vi "Drive Controller.vi"(8 "error in":errorcluster) -> ()   [LabVIEW 2019]
doc: "This VI executes continuously carrying out the current operation and responding to updates or new operation requests. It will often contain the timing or control code that is difficult to place directly in TeleOp. This VI generally opens all sensors and motors and isolates the rest of the robot code from knowing implementation details of how the operations are carried out."
uses:
  <vilib>/Rock Robotics/WPI/Framework/Completion Status.ctl
  Drive Setpoints.ctl
  Drive Operations.ctl
  <vilib>/Rock Robotics/WPI/ThirdParty/Phoenix-LabVIEW/Motor Controller/Controls/CTRE_Phoenix_MotorControl_ControlMode.ctl
  <vilib>/Rock Robotics/WPI/ThirdParty/Phoenix-LabVIEW/Motor Controller/Get/CTRE_Phoenix_MotorController_GetSelectedSensorData.vi
  <vilib>/Rock Robotics/WPI/SafetyOutput/WPI_SafetyOutputConfigMenu.ctl
  <vilib>/Rock Robotics/WPI/RobotDrive/WPI_RobotDriveOpen2MotorWithExistingMotors.vi
panel:
  in  "Interactive Values":T1
  in  "Buttons":cluster{"Execute Cmd":bool, "Abort Cmd":bool}
  out "Command Timing":cluster{"Start Time (ms)":u32, "Iterations":i32}
  out "Status":T3
  out "Current\nCmd":string
  # "Tip: The graph shows the motor setpoints. It may also be helpful to observe inputs and sensor values.\nYou may also want to display tuning or debugging controls."
  # "Interactive Command: You may fill in the settings for a command\nand schedule it with the Execute button. You can observe and abort\nany command while fine tuning the code for the controller."
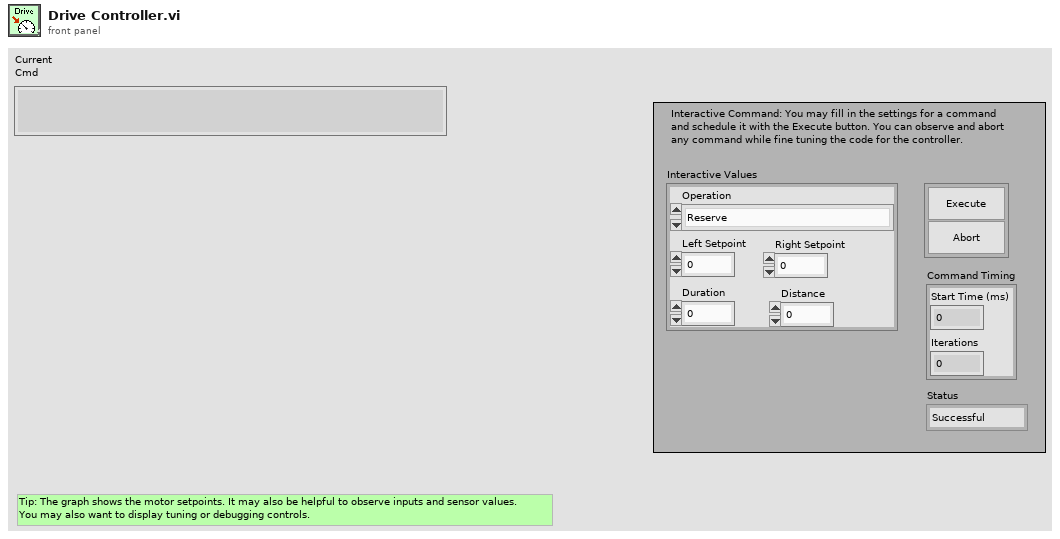
[diagram p1: front panel]
types:
  T1 = typedef "Drive Setpoints.ctl" = cluster{"Operation":T2, "Left Setpoint":dbl, "Right Setpoint":dbl, "Duration":dbl, "Distance":dbl}
  T2 = typedef "Drive Operations.ctl" = enum16{"Reserve", "Read Current", "Immediate", "Drive for Time", "Drive for Distance", "Turn angle"}
  T3 = typedef "Completion Status.ctl" = enum16{"Successful", "Aborted", "Incomplete"}
  T4 = typedef "WPI_SafetyOutputConfigMenu.ctl" = enum16{"Enable", "Disable"}
  T5 = typedef "WPI_MotorControlDeviceRef.ctl" = cluster{"DeviceStatus":errorcluster, "Type":T6, "PWM":cluster{"PWM Channel":T7, "DeadBand":T8}, "CAN":cluster{"Device Number":u8, "SetOutput VI Ref":variant, "GetOutput VI Ref":variant, "Enable VI Ref":variant, "Disable VI Ref":variant, "Data":variant}, "Invert":bool, "DIO PWM":cluster{"PWM \"Enable\" Channel":T7, "DIOChannel":T9, "PWM Rate":dbl}}
  T6 = typedef "WPI_MotorControlType.ctl" = enum16{"PWM", "CAN", "DIO PWM"}
  T7 = typedef "FPGA_DIOPWMChannel.ctl" = enum8{"PWM 0", "PWM 1", "PWM 2", "PWM 3", "PWM 4", "PWM 5", "PWM 6", "PWM 7", "PWM 8", "PWM 9", "PWM MXP 0", "PWM MXP 1", "PWM MXP 2", "PWM MXP 3", "PWM MXP 4", "PWM MXP 5", "PWM MXP 6", "PWM MXP 7", "PWM MXP 8", "PWM MXP 9", "Invalid"}
  T8 = typedef "WPI_PWMDeadband.ctl" = cluster{"Name":string, "maxPositivePwm":i32, "minPositivePwm":i32, "centerPwm":i32, "maxNegativePwm":i32, "minNegativePwm":i32, "angularRange":u16}
  T9 = typedef "FPGA_DIOChannel.ctl" = enum8{"DIO 0", "DIO 1", "DIO 2", "DIO 3", "DIO 4", "DIO 5", "DIO 6", "DIO 7", "DIO 8", "DIO 9", "DIO MXP 0", "DIO MXP 1", "DIO MXP 2", "DIO MXP 3", "DIO MXP 4", "DIO MXP 5", "DIO MXP 6", "DIO MXP 7", "DIO MXP 8", "DIO MXP 9", "DIO MXP 10", "DIO MXP 11", "DIO MXP 12", "DIO MXP 13", "DIO MXP 14", "DIO MXP 15", "SPI Port CS1", "SPI Port CS2", "SPI Port CS3", "SPI Port MISO", "SPI Port MOSI", "Invalid"}
  T10 = typedef "WPI_RobotDriveDevRef.ctl" = cluster{"DevStatus":errorcluster, "Motors[]":T5[], "Square Inputs":bool, "Max Output":dbl}
  T11 = enum16{"FollowerType_PercentOutput", "FollowerType_AuxOutput1"}
  T12 = typedef "Command Status Info.ctl" = cluster{"Name":string, "Status":T3, "notifier out":T13}
  T13 = typedef "Completion Notifier.ctl" = refnum<notifier>
  T14 = cluster{"SubSystem Data":T1, cluster{"Start Time (ms)":u32, "Iterations":i32}, cluster{"Command Info":T12, "Description":string, "Default Command":T1, "queue out":refnum<queue>, "Subsystem Name":string}}
  T15 = typedef "CTRE_Phoenix_MotorControl_ControlMode.ctl" = u16
  T16 = cluster{"SubSystem Data":T1, cluster{"Start Time (ms)":u32, "Iterations":i32}, "Default Command Arguments":cluster{"Command Info":T12, "Description":string, "Default Command":T1, "queue out":refnum<queue>, "Subsystem Name":string}}
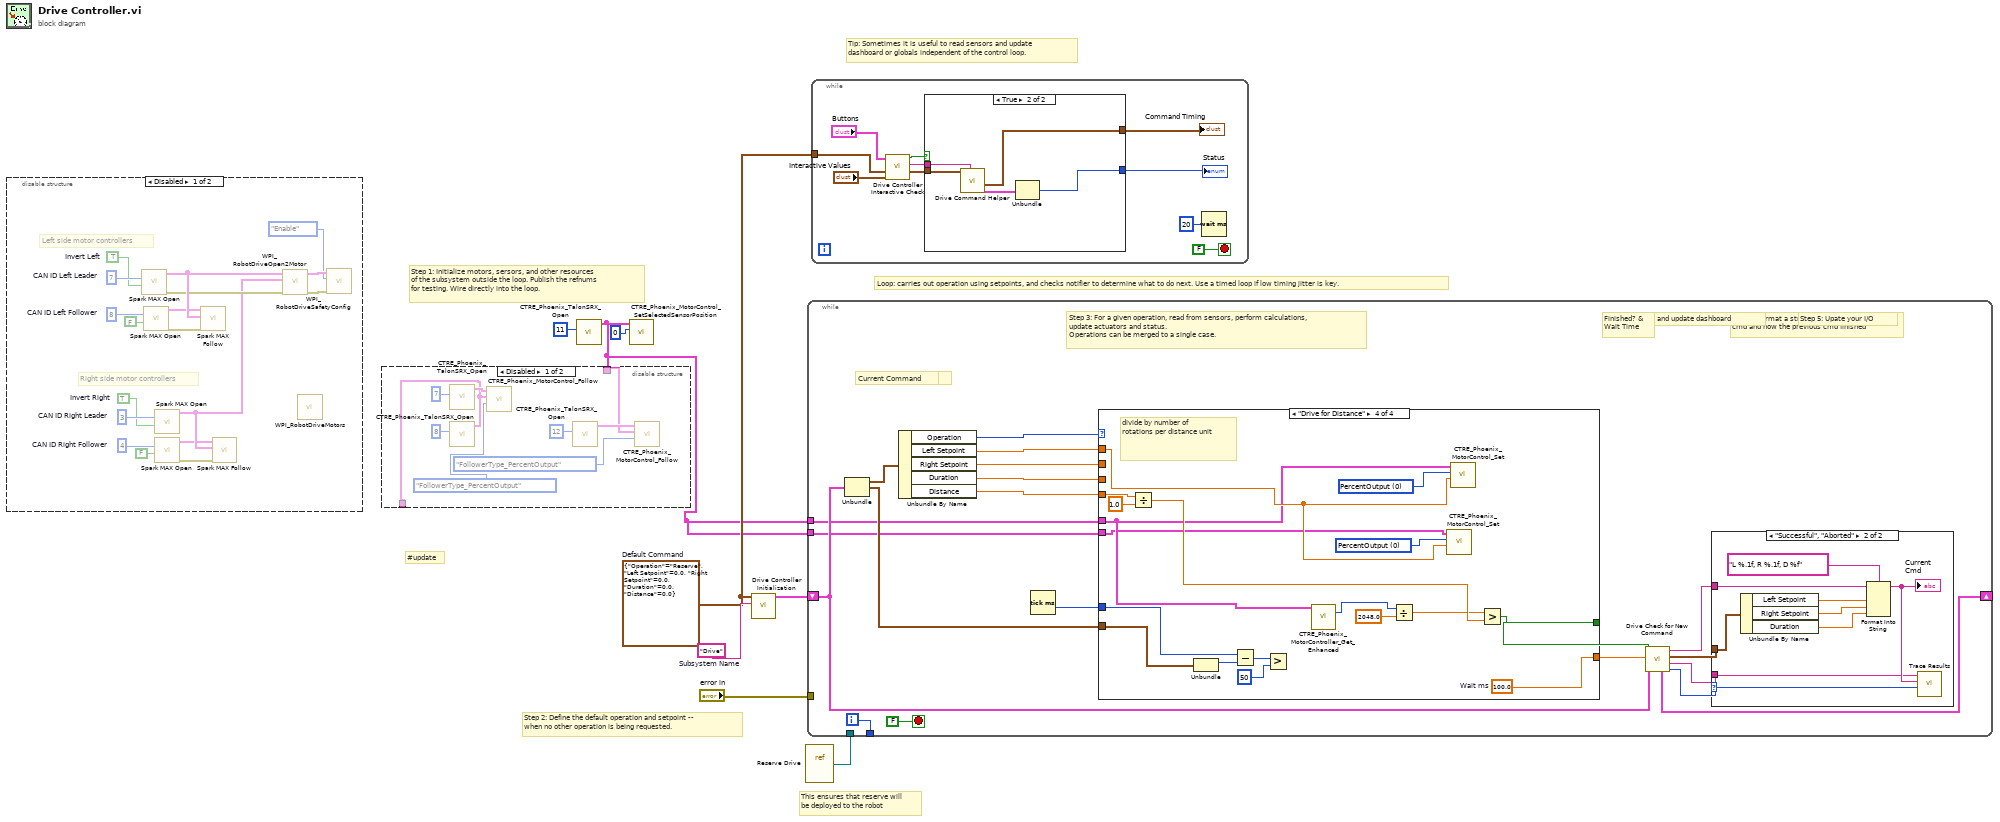
[diagram p0: block diagram]
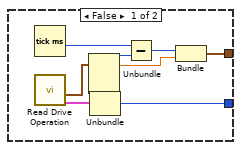
[diagram p4: hidden frame]
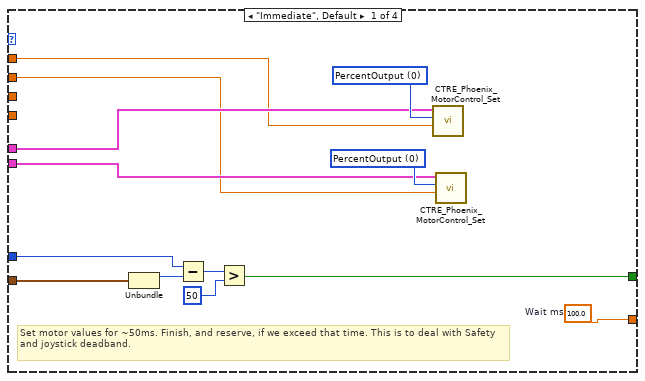
[diagram p6: hidden frame]
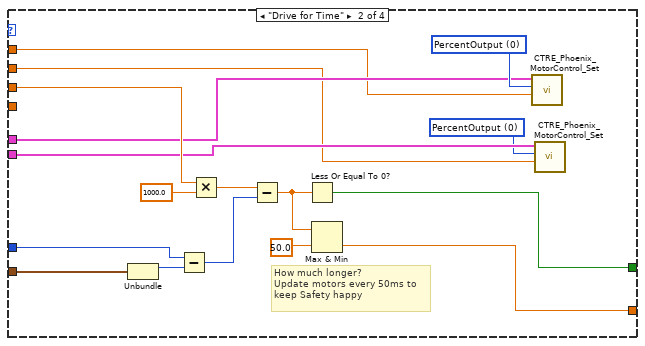
[diagram p7: hidden frame]
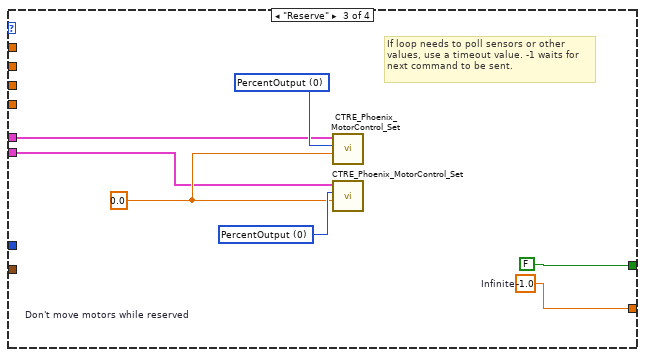
[diagram p8: hidden frame]
diagram:
  w4 = T1 {"Operation"=enum."Reserve", "Left Setpoint"=0.0, "Right Setpoint"=0.0, "Duration"=0.0, "Distance"=0.0}  # Default Command
  w8 = "Drive"  # Subsystem Name
  # "#update"
  # "This ensures that reserve will\nbe deployed to the robot"
  # "Tip: Sometimes it is useful to read sensors and update\ndashboard or globals independent of the control loop."
  # "Step 2: Define the default operation and setpoint --\nwhen no other operation is being requested."
  # "Step 1: Initialize motors, sersors, and other resources\nof the subsystem outside the loop. Publish the refnums\nfor testing. Wire directly into the loop."
  # "Loop: carries out operation using setpoints, and checks notifier to determine what to do next. Use a timed loop if low timing jitter is key."
  n1 = disable-structure shown="Disabled" {
    frame Disabled {
      w15 = TRUE  # Invert Left
      w14 = TRUE  # Invert Right
      w20 = u8 3  # CAN ID Right Leader
      w19 = u8 4  # CAN ID Right Follower
      w26 = u8 7  # CAN ID Left Leader
      w27 = u8 8  # CAN ID Left Follower
      # "Right side motor controllers"
      # "Left side motor controllers"
      n2 = call <vilib>:"Spark MAX Open.vi"("Invert"=w15, "Device Number"=w26) -> ("error out"=w24:errorcluster, "MotorControlDeviceRef"=w25:T5)  [unwired: 8 in]
      n3 = call <vilib>:"Spark MAX Open.vi"("Invert"=FALSE, "Device Number"=w27) -> ("error out"=w22:errorcluster, "MotorControlDeviceRef"=w23:T5)  [unwired: 8 in]
      n4 = call <vilib>:"Spark MAX Open.vi"("Invert"=w14, "Device Number"=w20) -> ("MotorControlDeviceRef"=w11:T5)  [unwired: 8 in, 1 out]
      n5 = call <vilib>:"Spark MAX Open.vi"("Invert"=FALSE, "Device Number"=w19) -> ("error out"=w21:errorcluster, "MotorControlDeviceRef"=w9:T5)  [unwired: 8 in]
      n6 = call <vilib>:"Spark MAX Follow.vi"("error in (no error)"=w22, "Master Controller"=w25, "MotorControlDeviceRef"=w23) -> ()  [unwired: 7 in, 2 out]
      n7 = call <vilib>:"Spark MAX Follow.vi"("error in (no error)"=w21, "Master Controller"=w11, "MotorControlDeviceRef"=w9) -> ()  [unwired: 7 in, 2 out]
      n8 = call-poly <vilib>:"WPI_RobotDriveOpen2Motor.vi"("error in (no error)"=w24, "Right Motor Dev Ref"=w11, "Left Motor Dev Ref"=w25) -> ("error out"=w17:errorcluster, "RobotDriveDevRef"=w18:T10)  [unwired: 7 in]
      n9 = call <vilib>:"WPI_RobotDriveMotors.vi"() -> ()  [unwired: 4 in, 8 out]
      n10 = call <vilib>:"WPI_RobotDriveSafetyConfig.vi"("error in (no error)"=w17, "mode"=WPI_SafetyOutputConfigMenu."Enable", "RobotDriveDevRef"=w18) -> ("RobotDriveDevRef"=w10:T10)  [unwired: 7 in, 1 out]
    }
    frame Enabled {
    }
  }
  n11 = call <vilib>:"CTRE_Phoenix_TalonSRX_Open.vi"("Device Number"=u8 11) -> ("CAN Talon SRX Ref"=w1:T5)  [unwired: 9 in, 1 out]
  n12 = disable-structure shown="Disabled" {
    disable-tunnel: [w30 _] -> _
    disable-tunnel: w1 -> [w29 _]
    frame Disabled {
      n13 = call <vilib>:"CTRE_Phoenix_TalonSRX_Open.vi"("Device Number"=u8 7) -> ("CAN Talon SRX Ref"=w31:T5)  [unwired: 9 in, 1 out]
      n14 = call <vilib>:"CTRE_Phoenix_TalonSRX_Open.vi"("Device Number"=u8 8) -> ("CAN Talon SRX Ref"=w30:T5)  [unwired: 9 in, 1 out]
      n15 = call <vilib>:"CTRE_Phoenix_MotorControl_Follow.vi"("FollowerType"=T11."FollowerType_PercentOutput", "Master Controller to Follow"=w30, "PhoenixMotorControlDevRef"=w31) -> ()  [unwired: 7 in, 2 out]
      n16 = call <vilib>:"CTRE_Phoenix_TalonSRX_Open.vi"("Device Number"=u8 12) -> ("CAN Talon SRX Ref"=w36:T5)  [unwired: 9 in, 1 out]
      n17 = call <vilib>:"CTRE_Phoenix_MotorControl_Follow.vi"("FollowerType"=T11."FollowerType_PercentOutput", "Master Controller to Follow"=w29, "PhoenixMotorControlDevRef"=w36) -> ()  [unwired: 7 in, 2 out]
    }
    frame Enabled {
    }
  }
  n18 = call <vilib>:"CTRE_Phoenix_MotorControl_SetSelectedSensorPosition.vi"("New Sensor Position"=0, "PhoenixMotorControlDevRef"=w1) -> ()  [unwired: 8 in, 2 out]
  n19 = call "Drive Controller Initialization.vi"("Subsystem Name"=w8, "Default Command"=w4) -> ("Current Command"=w6:T14)  [unwired: 9 in]
  n20 = vi-ref "Reserve Drive.vi"() -> (w5:refnum<vi>)
  n21 = while {
    shift-right: [w47] -> _
    shift-left: w6 -> [w40]
    tunnel: [w55] -> _
    tunnel: "error in" -> [_]
    tunnel: w5 -> [_]
    tunnel: w1 -> [w38]
    tunnel: w1 -> [w37]
    i -> [w55]
    stop <- FALSE stop-if-true
    # "Step 5: Upate your I/O"
    # "Step 4: Format a string to describe this\ncmd and how the previous cmd finished"
    # "Current Command"
    # "Update motors and update dashboard"
    # "Access Cmd setpoints"
    # "Finished? &\nWait Time"
    # "Step 3: For a given operation, read from sensors, perform calculations,\nupdate actuators and status.\nOperations can be merged to a single case."
    n22 = Unbundle(w40) -> ("SubSystem Data"=w54:T1, w41:cluster{"Start Time (ms)":u32, "Iterations":i32})  [unwired: 1 out]
    n23 = Unbundle By Name(w54) -> ("Operation"=w53:T2, "Left Setpoint"=w52:dbl, "Right Setpoint"=w51:dbl, "Duration"=w50:dbl, "Distance"=w39:dbl)
    n24 = Tick Count (ms)() -> (millisecond timer value=w49:u32)
    n25 = case shown="\"Drive for Distance\"" w53 {
      tunnel: [w78 w85 w102 w115] -> w46
      tunnel: [w73 w90 FALSE ("ignore previous (F)") w105] -> w45
      tunnel: w41 -> [w72 w92 _ w114]
      tunnel: w52 -> [w67 w81 _ w111]
      tunnel: w51 -> [w66 w80 _ _]
      tunnel: w50 -> [_ w89 _ _]
      tunnel: w49 -> [w74 w88 _ w112]
      tunnel: w39 -> [_ _ _ w120]
      tunnel: w38 -> [w68 w82 w96 w103]
      tunnel: w37 -> [w69 w83 w97 w104]
      frame "Immediate", Default {
        w70 = T15 0 items=["PercentOutput"=0, "Position"=1, "Velocity"=2, "Current"=3, "Follower"=5, "MotionProfile"=6, "MotionMagic"=7, "MotionProfileArc"=10, "Disabled"=15] ("Control Mode")
        w71 = T15 0 items=["PercentOutput"=0, "Position"=1, "Velocity"=2, "Current"=3, "Follower"=5, "MotionProfile"=6, "MotionMagic"=7, "MotionProfileArc"=10, "Disabled"=15] ("Control Mode")
        w78 = 100.0  # Wait ms
        # "Set motor values for ~50ms. Finish, and reserve, if we exceed that time. This is to deal with Safety and joystick deadband."
        n26 = Unbundle(w72) -> ("Start Time (ms)"=w75:u32)  [unwired: 1 out]
        n27 = Subtract(x=w74, y=w75) -> (x-y=w76:u32)
        n28 = Greater?(x=w76, y=u8 50 ("Left Motor")) -> (0:w73:bool)
        n29 = call <vilib>:"CTRE_Phoenix_MotorControl_Set.vi"("Output"=w67, "Control Mode"=w71, "PhoenixMotorControlDevRef"=w69) -> ()  [unwired: 7 in, 2 out]
        n30 = call <vilib>:"CTRE_Phoenix_MotorControl_Set.vi"("Output"=w66, "Control Mode"=w70, "PhoenixMotorControlDevRef"=w68) -> ()  [unwired: 7 in, 2 out]
      }
      frame "Drive for Time" {
        w79 = T15 0 items=["PercentOutput"=0, "Position"=1, "Velocity"=2, "Current"=3, "Follower"=5, "MotionProfile"=6, "MotionMagic"=7, "MotionProfileArc"=10, "Disabled"=15] ("Control Mode")
        w84 = T15 0 items=["PercentOutput"=0, "Position"=1, "Velocity"=2, "Current"=3, "Follower"=5, "MotionProfile"=6, "MotionMagic"=7, "MotionProfileArc"=10, "Disabled"=15] ("Control Mode")
        # "How much longer?\nUpdate motors every 50ms to\nkeep Safety happy"
        n31 = Unbundle(w92) -> ("Start Time (ms)"=w91:u32)  [unwired: 1 out]
        n32 = Subtract(x=w88, y=w91) -> (x-y=w95:u32)
        n33 = Multiply(x=w89, y=1000.0) -> (x*y=w94:dbl)
        n34 = Subtract(x=w94, y=w95) -> (x-y=w87:dbl)
        n35 = Less Or Equal To 0?(x=w87) -> (x <= 0?=w90:bool)
        n36 = Max & Min(x=w87, y=50.0) -> (min(x,y)=w85:dbl)  [unwired: 1 out]
        n37 = call <vilib>:"CTRE_Phoenix_MotorControl_Set.vi"("Output"=w81, "Control Mode"=w84, "PhoenixMotorControlDevRef"=w83) -> ()  [unwired: 7 in, 2 out]
        n38 = call <vilib>:"CTRE_Phoenix_MotorControl_Set.vi"("Output"=w80, "Control Mode"=w79, "PhoenixMotorControlDevRef"=w82) -> ()  [unwired: 7 in, 2 out]
      }
      frame "Reserve" {
        w99 = T15 0 items=["PercentOutput"=0, "Position"=1, "Velocity"=2, "Current"=3, "Follower"=5, "MotionProfile"=6, "MotionMagic"=7, "MotionProfileArc"=10, "Disabled"=15] ("Control Mode")
        w100 = T15 0 items=["PercentOutput"=0, "Position"=1, "Velocity"=2, "Current"=3, "Follower"=5, "MotionProfile"=6, "MotionMagic"=7, "MotionProfileArc"=10, "Disabled"=15] ("Control Mode")
        w98 = 0.0  # Don't move motors while reserved
        w102 = -1.0  # Infinite
        # "If loop needs to poll sensors or other\nvalues, use a timeout value. -1 waits for\nnext command to be sent."
        n39 = call <vilib>:"CTRE_Phoenix_MotorControl_Set.vi"("Output"=w98, "Control Mode"=w100, "PhoenixMotorControlDevRef"=w97) -> ()  [unwired: 7 in, 2 out]
        n40 = call <vilib>:"CTRE_Phoenix_MotorControl_Set.vi"("Output"=w98, "Control Mode"=w99, "PhoenixMotorControlDevRef"=w96) -> ()  [unwired: 7 in, 2 out]
      }
      frame "Drive for Distance" {
        w107 = T15 0 items=["PercentOutput"=0, "Position"=1, "Velocity"=2, "Current"=3, "Follower"=5, "MotionProfile"=6, "MotionMagic"=7, "MotionProfileArc"=10, "Disabled"=15] ("Control Mode")
        w110 = T15 0 items=["PercentOutput"=0, "Position"=1, "Velocity"=2, "Current"=3, "Follower"=5, "MotionProfile"=6, "MotionMagic"=7, "MotionProfileArc"=10, "Disabled"=15] ("Control Mode")
        w115 = 100.0  # Wait ms
        # "divide by number of rotations per distance unit"
        n41 = Divide(x=w120, y=1.0) -> (x/y=w119:dbl)
        n42 = Unbundle(w114) -> ("Start Time (ms)"=w113:u32)  [unwired: 1 out]
        n43 = Subtract(x=w112, y=w113) -> (x-y=w116:u32)
        n44 = Greater?(x=w116, y=u8 50 ("Left Motor")) -> ()  [unwired: 1 out]
        n45 = call-poly <vilib>:"CTRE_Phoenix_MotorController_Get_Enhanced.vi"("PhoenixMotorControlDevRef"=w104) -> ("Position (Raw Sensor Units)"=w106:i32)  [unwired: 11 in, 3 out]
        n46 = Divide(x=w106, y=2048.0) -> (x/y=w109:dbl)
        n47 = call <vilib>:"CTRE_Phoenix_MotorControl_Set.vi"("Output"=w111, "Control Mode"=w110, "PhoenixMotorControlDevRef"=w103) -> ()  [unwired: 7 in, 2 out]
        n48 = call <vilib>:"CTRE_Phoenix_MotorControl_Set.vi"("Output"=w111, "Control Mode"=w107, "PhoenixMotorControlDevRef"=w104) -> ()  [unwired: 7 in, 2 out]
        n49 = Greater?(x=w109, y=w119) -> (0:w105:bool)
      }
    }
    n50 = call "Drive Check for New Command.vi"("input cluster"=w40, "Wait time (ms)"=w46, "Finished?"=w45) -> ("Completion"=w48:T3, "Subsystem Name"=w42:string, "Current Command"=w43:T1, "Initial Trace String"=w44:string, "Next Command"=w47:T16)  [unwired: 4 in]
    n51 = case shown="\"Successful\", \"Aborted\"" w48 {
      selector: w48 -> [_ w65]
      tunnel: w44 -> [_ w60]
      tunnel: w43 -> [_ w61]
      tunnel: w42 -> [_ w57]
      frame "Incomplete", Default {
        # "Continuing current command"
      }
      frame "Successful", "Aborted" {
        # "Report and setup for next command"
        n52 = Unbundle By Name(w61) -> ("Left Setpoint"=w63:dbl, "Right Setpoint"=w64:dbl, "Duration"=w58:dbl)
        n53 = Format Into String(format string="L %.1f, R %.1f, D %f", initial string=w60, w63, w64, w58) -> (resulting string=w59:string)  [unwired: 1 in, 1 out]
        "Current\nCmd" <- w59
        n54 = call <vilib>:"Trace Results.vi"("Status of previous command"=w65, "Description"=w59, "Subsystem"=w57) -> ()  [unwired: 9 in]
      }
    }
  }
  n55 = while {
    tunnel: w4 -> [w122]
    stop <- FALSE stop-if-true
    n56 = call "Drive Controller Interactive Check.vi"("Interactive Command In"="Interactive Values", "Default Command"=w122, "Buttons"="Buttons") -> ("Interactive Command Out"=w124:T1, "Trace String"=w125:string, "Schedule"=w126:bool)  [unwired: 6 in]
    n57 = case shown="True" w126 {
      tunnel: [w135 w143] -> w127
      tunnel: [w134 w139] -> w128
      tunnel: w125 -> [_ w141]
      tunnel: w124 -> [_ w140]
      frame False {
        n58 = Tick Count (ms)() -> (millisecond timer value=w138:u32)
        n59 = call "Read Drive Operation.vi"() -> ("Command Info"=w132:T12, "SubSystem Data"=w131:T1)  [unwired: 9 in, 1 out]
        n60 = Unbundle(w131) -> ("Operation"=w136:T2, "Left Setpoint"=w133:dbl)  [unwired: 3 out]
        n61 = Unbundle(w132) -> ("Status"=w135:T3)  [unwired: 2 out]
        n62 = Subtract(x=w138, y=w136) -> (x-y=w137:u32)
        n63 = Bundle(w137, "Left Setpoint"=w133) -> (w134:cluster{u32, "Left Setpoint":dbl})  [unwired: 1 in]
      }
      frame True {
        n64 = call "Drive Command Helper.vi"("Description"=w141, "SubSystem Data"=w140) -> ("Command Info Out"=w142:T12, "Command Timing"=w139:cluster{"Start Time (ms)":u32, "Iterations":i32})  [unwired: 7 in, 1 out]
        n65 = Unbundle(w142) -> ("Status"=w143:T3)  [unwired: 2 out]
      }
    }
    "Status" <- w127
    "Command Timing" <- w128
    n66 = Wait (ms)(milliseconds to wait=u32 20) -> ()  [unwired: 1 out]
  }
